vi "TestInitialize.vi"(8 "error in (no error)":errorcluster) -> (0 "error out":errorcluster)   [LabVIEW 2017]
uses:
  src/API/JKI Simple Localization.lvlib
  <vilib>/addons/_JKI Toolkits/Caraya/classes/Test/Test.lvclass
  <vilib>/addons/_JKI Toolkits/Caraya/classes/Assert/Assert.lvclass
panel:
  # "See block diagram for unit tests of Initialize.vi"
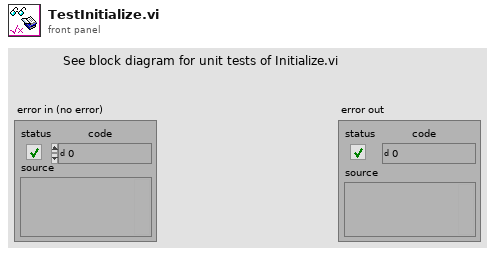
[diagram p1: front panel]
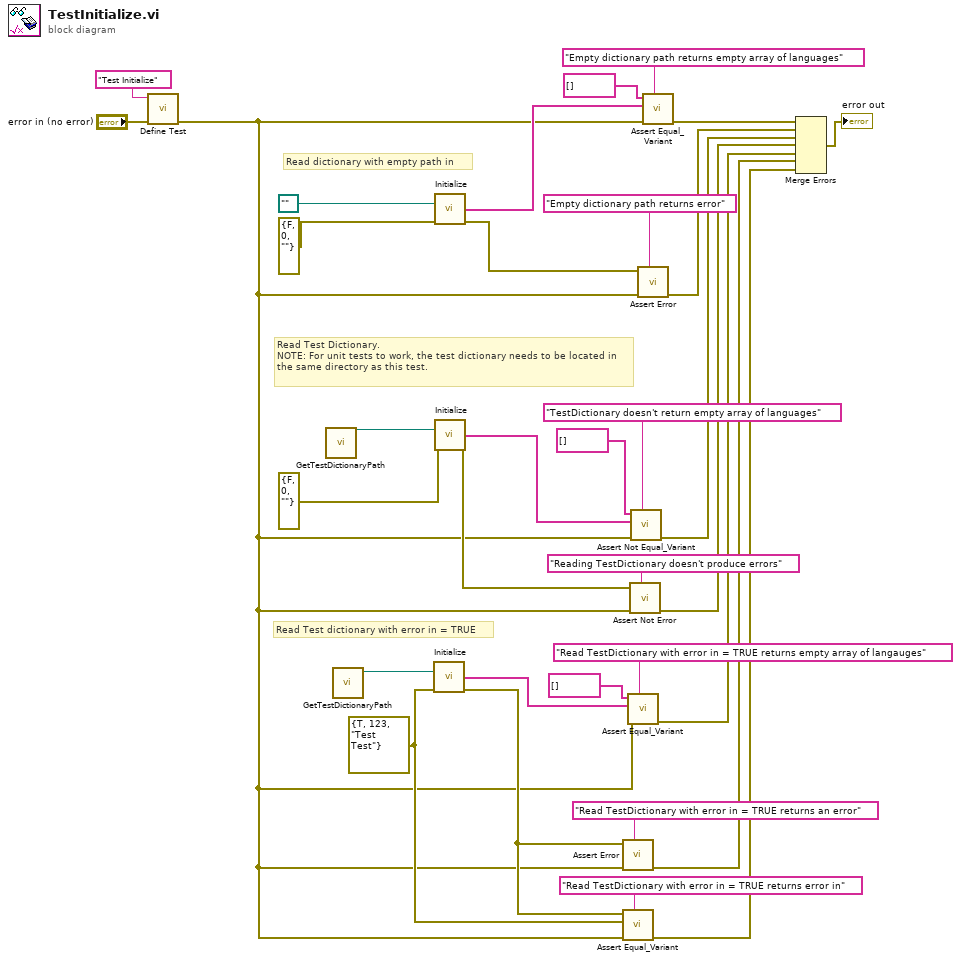
[diagram p0: block diagram]
diagram:
  w14 = errorcluster {"status"=TRUE, "code"=123, "source"="Test Test"} ("error in")
  # "Read Test dictionary with error in = TRUE"
  # "Read dictionary with empty path in"
  # "Read Test Dictionary. \nNOTE: For unit tests to work, the test dictionary needs to be located in the same directory as this test."
  n1 = call <vilib>:"Define Test.vi"("error in (no error)"="error in (no error)", "Label (VI Title)"="Test Initialize") -> ("error out"=w13:errorcluster)  [unwired: 9 in]
  n2 = call "GetTestDictionaryPath.vi"() -> ("Test Dictionary Path"=w26:path)  [unwired: 11 in]
  n3 = call "GetTestDictionaryPath.vi"() -> ("Test Dictionary Path"=w1:path)  [unwired: 11 in]
  n4 = call "Initialize.vi"("Dictionary File Path"=w1, "error in"=w14) -> ("Languages"=w16:string[], "error out"=w15:errorcluster)  [unwired: 10 in, 2 out]
  n5 = call "Initialize.vi"("Dictionary File Path"=path "", "error in"=errorcluster {"status"=FALSE, "code"=0, "source"=""}) -> ("Languages"=w30:string[], "error out"=w31:errorcluster)  [unwired: 10 in, 2 out]
  n6 = call "Initialize.vi"("Dictionary File Path"=w26, "error in"=errorcluster {"status"=FALSE, "code"=0, "source"=""}) -> ("Languages"=w23:string[], "error out"=w21:errorcluster)  [unwired: 10 in, 2 out]
  n7 = call <vilib>:"Assert Error.vi"("Label"="Read TestDictionary with error in = TRUE returns an error", "error in (no error)"=w13, "Error?"=w15) -> ("error out"=w3:errorcluster)  [unwired: 8 in]
  n8 = call <vilib>:"Assert Equal_Variant.vi"("Label"="Read TestDictionary with error in = TRUE returns error in", "error in (no error)"=w13, "Y"=w14, "X"=w15) -> ("error out"=w2:errorcluster)  [unwired: 7 in]
  n9 = call <vilib>:"Assert Equal_Variant.vi"("Label"="Read TestDictionary with error in = TRUE returns empty array of langauges", "error in (no error)"=w13, "Y"=w16, "X"=string[] []) -> ("error out"=w4:errorcluster)  [unwired: 7 in]
  n10 = call <vilib>:"Assert Not Error.vi"("Label"="Reading TestDictionary doesn't produce errors", "error in (no error)"=w13, "Not Error?"=w21) -> ("error out"=w5:errorcluster)  [unwired: 8 in]
  n11 = call <vilib>:"Assert Not Equal_Variant.vi"("Label"="TestDictionary doesn't return empty array of languages", "error in (no error)"=w13, "Y"=w23, "X"=string[] []) -> ("error out"=w6:errorcluster)  [unwired: 7 in]
  n12 = call <vilib>:"Assert Error.vi"("Label"="Empty dictionary path returns error", "error in (no error)"=w13, "Error?"=w31) -> ("error out"=w7:errorcluster)  [unwired: 8 in]
  n13 = call <vilib>:"Assert Equal_Variant.vi"("Label"="Empty dictionary path returns empty array of languages", "error in (no error)"=w13, "Y"=w30, "X"=string[] []) -> ("error out"=w10:errorcluster)  [unwired: 7 in]
  n14 = Merge Errors(w10, w7, w6, w5, w4, w3, w2) -> (→"error out":errorcluster)
